vi "CSM - Query CSM VI Ref By API String.vi"(6 "Response Timeout(5000ms)":i32=5000, 7 "Current Module(\"\" to generate a ID)":string, 8 "Error In (no error)":errorcluster, 9 "Target Module":string="A") -> (0 "error out":errorcluster, 3 "CSM VI Ref":refnum<vi>)   [LabVIEW 2017, in "API String Arguments Support.lvlib"]
doc: "This VI is oblselete. Please use \"CSM - Module VI Reference.vi\" instead."
uses:
  API String Arguments Support.lvlib
  <userlib>/_NEVSTOP/Communicable State Machine(CSM)/Communicable State Machine.lvlib
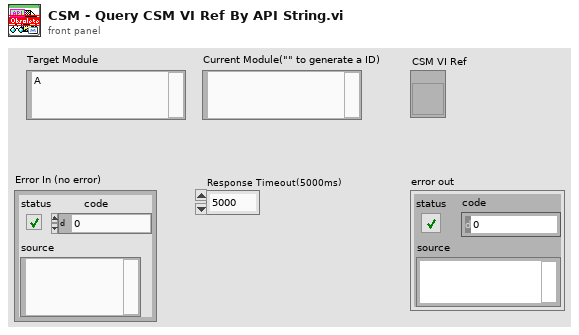
[diagram p1: front panel]
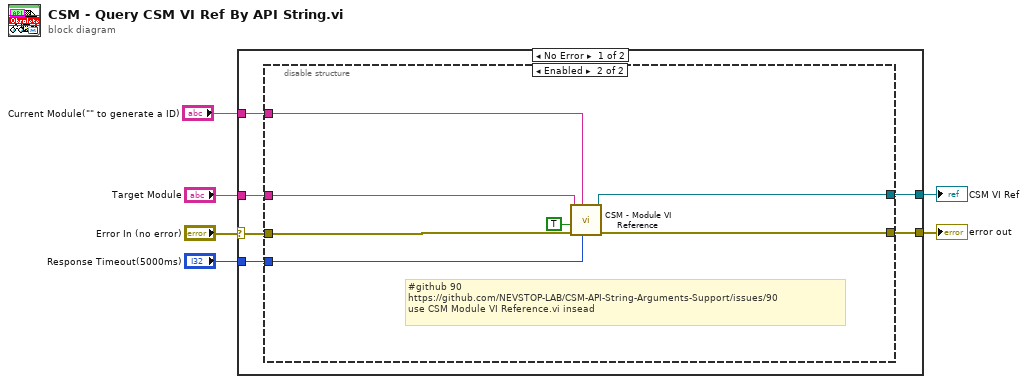
[diagram p0: block diagram]
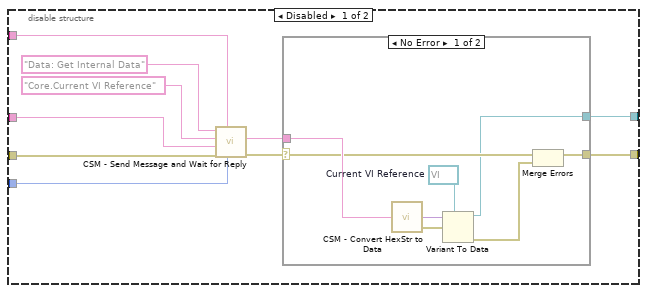
[diagram p2: hidden frame]
diagram:
  n1 = case shown="No Error" "Error In (no error)" {
    selector: "Error In (no error)" -> [w10 w39]
    tunnel: "Response Timeout(5000ms)" -> [w12 _]
    tunnel: [w11 w39] -> w5
    tunnel: [w9 _] -> w3
    tunnel: "Target Module" -> [w8 _]
    tunnel: "Current Module(\"\" to generate a ID)" -> [w7 _]
    frame No Error {
      n2 = disable-structure shown="Enabled" {
        disable-tunnel: w12 -> [w21 w32]
        disable-tunnel: [w18 w36] -> w11
        disable-tunnel: w10 -> [w17 w37]
        disable-tunnel: [w15 w34] -> w9
        disable-tunnel: w8 -> [w14 w35]
        disable-tunnel: w7 -> [w13 w33]
        frame Disabled {
          n3 = call <userlib>:"CSM - Send Message and Wait for Reply.vi"("Response Timeout(-2 using Global Settings)"=w21, "Current Module(\"\" to generate a ID)"=w13, "Error In (no error)"=w17, "Target Module"=w14, "Arguments (\"\")"="Core.Current VI Reference" ("Name(\"\" to use uuid)"), "State"="Data: Get Internal Data") -> ("error out"=w19:errorcluster, "Response"=w20:string)  [unwired: 3 in, 1 out]
          n4 = case shown="No Error" w19 {
            selector: w19 -> [w25 w31]
            tunnel: w20 -> [w30 _]
            tunnel: [w26 w31] -> w18
            tunnel: [w23 _] -> w15
            frame No Error {
              w27 = refnum<vi> refnum  # Current VI Reference
              n5 = call <userlib>:"CSM - Convert HexStr to Data.vi"("HEX String"=w30) -> ("Variant"=w28:variant, "error out"=w29:errorcluster)  [unwired: 7 in]
              n6 = Variant To Data(error in=w29, type=w27, Variant=w28) -> (data=w23:refnum<vi>, error out=w24:errorcluster)
              n7 = Merge Errors(w25, w24) -> (w26:errorcluster)
            }
            frame Error {
            }
          }
        }
        frame Enabled {
          # "#github 90\nhttps://github.com/NEVSTOP-LAB/CSM-API-String-Arguments-Support/issues/90\nuse CSM Module VI Reference.vi insead"
          n8 = call <userlib>:"CSM - Module VI Reference.vi"("Response Timeout(-2 using Global Settings)"=w32, "Current Module(\"\" to generate a ID)"=w33, "error in (no error)"=w37, "force?(F)"=TRUE, "CSM Name"=w35) -> ("error out"=w36:errorcluster, "CSM Module VIRef"=w34:refnum<vi>)  [unwired: 5 in]
        }
      }
    }
    frame Error {
    }
  }
  "error out" <- w5
  "CSM VI Ref" <- w3
